vi "Stop StateMachine.vi"(8 "error in (no error)":errorcluster, 11 "statemachine in":refnum<class "statemachine.lvclass">) -> (0 "error out":errorcluster, 3 "statemachine out":refnum<class "statemachine.lvclass">)   [LabVIEW 2020, in "eos.lvlib" / "statemachine.lvclass"]
uses:
  statemachine.lvclass
  states/shutting-down/shuttingDown.lvclass
  C:/Projects/LVOS/EngineeringOS/source/classes/states/shutting-down/shuttingDown.lvclass
  C:/Projects/LVOS/EngineeringOS/source/interfaces/state/state.lvclass
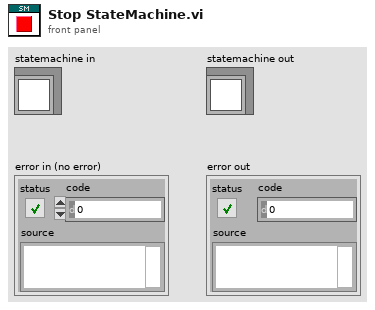
[diagram p1: front panel]
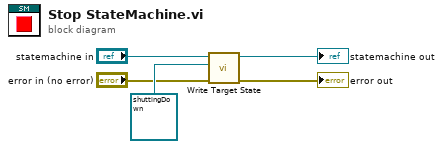
[diagram p0: block diagram]
diagram:
  n1 = call "Write Target State.vi"("Target State"=refnum<class "shuttingDown.lvclass"> refnum ("eos.lvlib:shuttingDown.lvclass"), "statemachine in"="statemachine in") -> ("statemachine out"=→"statemachine out":refnum<class "statemachine.lvclass">)  [unwired: 9 in]
  "error out" <- "error in (no error)"
